vi "Write COMM Address.vi"(8 "error in (no error)":errorcluster, 10 "COMM Address":string, 11 "DevInfo in":refnum<class "DevInfo.lvclass">) -> (0 "error out":errorcluster, 3 "DevInfo out":refnum<class "DevInfo.lvclass">)   [LabVIEW 2016, in "Hardware.lvlib" / "DevInfo.lvclass"]
uses:
  <userlib>/Common Components/Hardware/DevInfo/DevInfo.lvclass
  <userlib>/Common Components/Hardware/DevInfo/DevInfo.lvclass/DevInfo.ctl
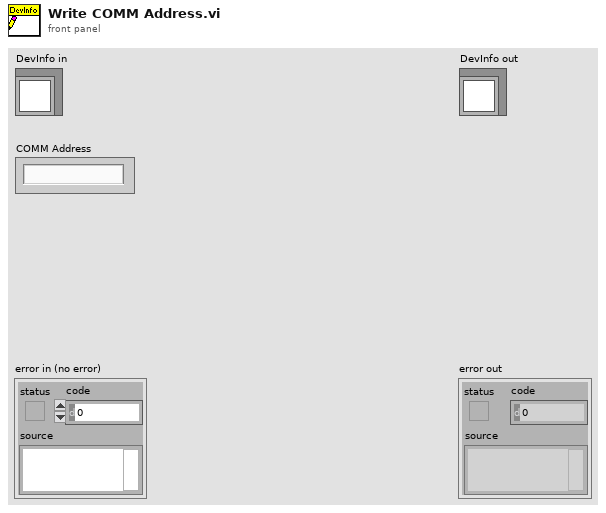
[diagram p1: front panel]
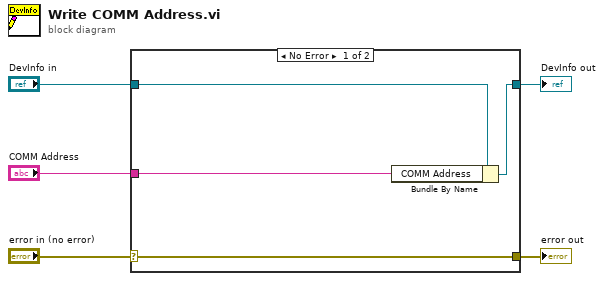
[diagram p0: block diagram]
diagram:
  n1 = case shown="No Error" "error in (no error)" {
    selector: "error in (no error)" -> [w9 w10]
    tunnel: [w9 w10] -> w4
    tunnel: [w7 w11] -> w2
    tunnel: "DevInfo in" -> [w8 w11]
    tunnel: "COMM Address" -> [w6 _]
    frame No Error {
      n2 = Bundle By Name(cluster=w8, "COMM Address"=w6) -> (w7:refnum<class "DevInfo.lvclass">)
    }
    frame Error {
    }
  }
  "error out" <- w4
  "DevInfo out" <- w2
